vi "Popup.vi"(8 "error in (no error)":errorcluster, 9 "Panel":refnum<class "Panel.lvclass">, 10 "String in":string, 11 "Boolean Data Type in":refnum<class "Boolean Data Type.lvclass">) -> (0 "error out":errorcluster, 2 "String out":string, 3 "Boolean Data Type out":refnum<class "Boolean Data Type.lvclass">)   [LabVIEW 2018, in "Boolean Data Type.lvclass"]
uses:
  Boolean Data Type.lvclass
  <vilib>/MGI/Panel Manager/Panel/Panel/Panel.lvclass
  Boolean Data Type.lvclass/Boolean Data Type.ctl
panel:
  in  "OK Button":bool
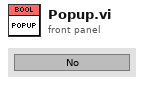
[diagram p1: front panel]
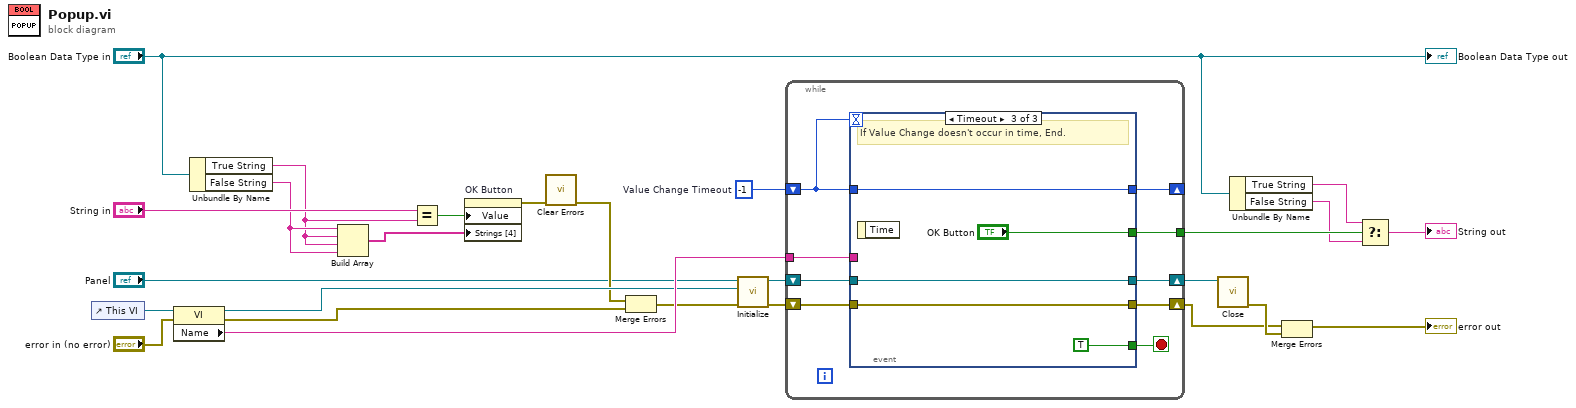
[diagram p0: block diagram]
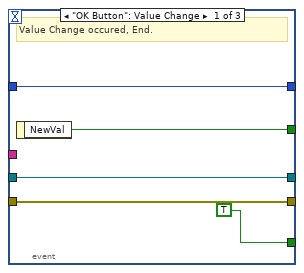
[diagram p2: hidden frame]
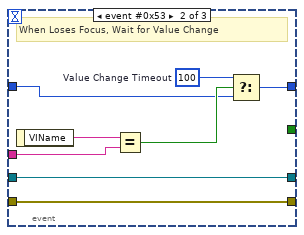
[diagram p3: hidden frame]
diagram:
  w25 = -1  # Value Change Timeout
  n1 = control-ref of="This VI"() -> (w20:refnum<vi>)
  n2 = property class="VI"(reference=w20, error in="error in (no error)") -> (reference out=w21:refnum<vi>, error out=w24:errorcluster, "Name"=w23:string)
  n3 = Unbundle By Name("Boolean Data Type in") -> ("True String"=w1:string, "False String"=w2:string)
  n4 = Build Array(w2, w1, w1, w2) -> (w11:string[])
  n5 = Equal?(x="String in", y=w1) -> (x = y?=w12:bool)
  n6 = property on="OK Button" class="Bool (strict)"("Value"=w12, "Strings [4]"=w11) -> (error out=w18:errorcluster)  [unwired: 2 in, 1 out]
  n7 = call <vilib>:"Clear Errors.vi"("error in (no error)"=w18) -> ("error out"=w19:errorcluster)  [unwired: 5 in, 1 out]
  n8 = Merge Errors(w19, w24) -> (w22:errorcluster)
  n9 = call <vilib>:"Initialize.vi"("error in (no error)"=w22, "VI Refnum"=w21, "Panel In"="Panel") -> ("error out"=w26:errorcluster, "Panel Out"=w14:refnum<class "Panel.lvclass">)  [unwired: 6 in, 1 out]
  n10 = while {
    shift-right: [w35] -> w16
    shift-left: w26 -> [w34]
    shift-right: [w32] -> w15
    shift-left: w14 -> [w31]
    tunnel: [w30] -> w8
    tunnel: w23 -> [w29]
    shift-right: [w27] -> _
    shift-left: w25 -> [w28]
    stop <- w33 stop-if-true
    n11 = event shown="[2] Timeout" {
      selector: _ -> [_ _ _]
      dyn-events: _ -> [_ _ _]
      timeout: w28 -> [_ _ _]
      tunnel: [w37 w46 w52] -> w35
      tunnel: w34 -> [w37 w46 w52]
      tunnel: [TRUE _ TRUE] -> w33
      tunnel: [w39 w45 w53] -> w32
      tunnel: w31 -> [w39 w45 w53]
      tunnel: [w38 _ "OK Button"] -> w30
      tunnel: w29 -> [_ w47 _]
      tunnel: w28 -> [w36 w42 w50]
      tunnel: [w36 w41 w50] -> w27
      event "OK Button": Value Change {
        # "Value Change occured, End."
        n12 = event-data() -> ("NewVal"=w38:bool)  [unwired: 1 in]
      }
      event event #0x53 {
        w43 = 100  # Value Change Timeout
        # "When Loses Focus, Wait for Value Change"
        n13 = event-data() -> ("VIName"=w48:string)  [unwired: 1 in]
        n14 = Equal?(x=w48, y=w47) -> (x = y?=w44:bool)
        n15 = Select(t=w43, s=w44, f=w42) -> (s? t:f=w41:i32)
      }
      event Timeout {
        # "If Value Change doesn't occur in time, End."
        n16 = event-data() -> ()  [unwired: 1 in, 1 out]
      }
    }
  }
  n17 = call-dynamic "Close.vi"("Panel In"=w15) -> ("Error Out"=w17:errorcluster)  [unwired: 10 in]
  n18 = Unbundle By Name("Boolean Data Type in") -> ("True String"=w5:string, "False String"=w4:string)
  n19 = Merge Errors(w16, w17) -> (→"error out":errorcluster)
  n20 = Select(t=w5, s=w8, f=w4) -> (s? t:f=→"String out":string)
  "Boolean Data Type out" <- "Boolean Data Type in"
